vi "Inter-trial delay.vi"(9 "error in":errorcluster, 11 "Trial index":i32) -> (1 "error out":errorcluster)   [LabVIEW 2020]
panel:
  in  "milliseconds to wait":u32=6
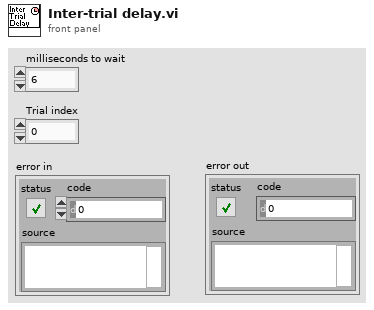
[diagram p1: front panel]
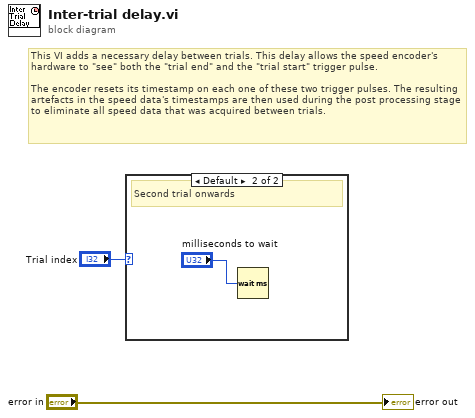
[diagram p0: block diagram]
diagram:
  # "This VI adds a necessary delay between trials. This delay allows the speed encoder's hardware to \"see\" both the \"trial end\" and the \"trial start\" trigger pulse.\n\nThe encoder resets its timestamp on each one of these two trigger pulses. The resulting artefacts in the speed data's timestamps are then used during the post processing stage to eliminate all speed data that was acquired between trials."
  n1 = case shown="Default" "Trial index" {
    frame 0 {
      # "First trial or Live imaging"
    }
    frame Default {
      # "Second trial onwards"
      n2 = Wait (ms)(milliseconds to wait="milliseconds to wait") -> ()  [unwired: 1 out]
    }
  }
  "error out" <- "error in"
